vi "selectHotLotNewLinked.vi"() -> (0 "data":string, 3 "Array":string[][](array[string]))   [LabVIEW 2012]
uses:
  <vilib>/addons/database/Auxilliary.llb/DB Tools Cursor Type.ctl
  <vilib>/addons/database/Connection.llb/DB Tools Open Connec (Path).vi
  <vilib>/addons/database/Connection.llb/Conn Execute.vi
  <vilib>/addons/database/Recordset.llb/Rec Fetch Recordset Data (R).vi
  <vilib>/addons/database/Recordset.llb/Rec Destroy - Connection.vi
  <vilib>/addons/database/_DB Variant To Data/Database Variant To Data.xnode
  <vilib>/addons/database/NI_Database_API.lvlib
panel:
  in  "Cluster":T1
  out "data 2":string
  out "error out":errorcluster
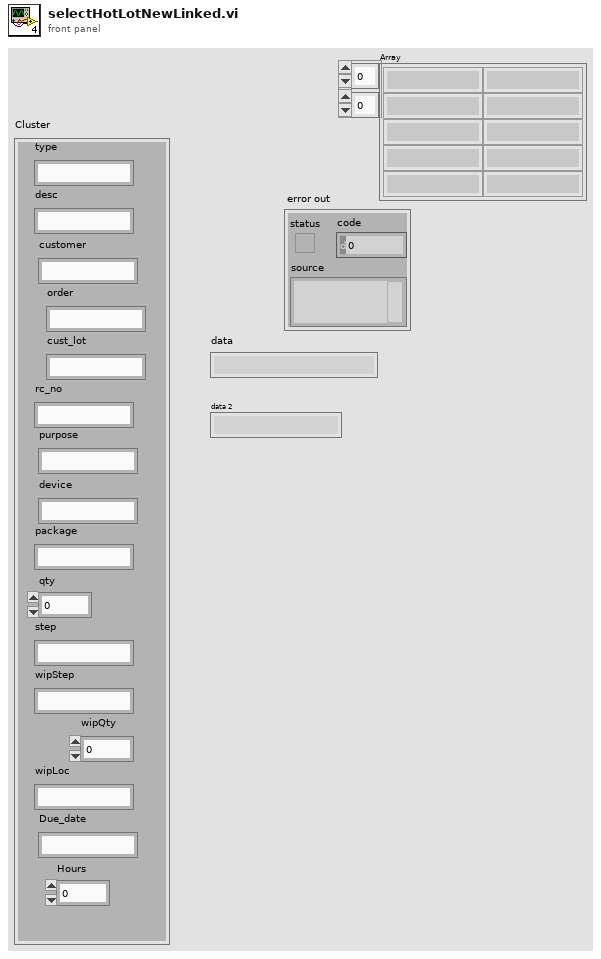
[diagram p1: front panel]
types:
  T1 = cluster{"type":string, "desc":string, "customer":string, "order":string, "cust_lot":string, "rc_no":string, "purpose":string, "device":string, "package":string, "qty":dbl, "step":string, "wipStep":string, "wipQty":dbl, "wipLoc":string, "Due_date":string, "Hours":dbl}
  T2 = typedef "NI_Database_API.lvlib/DB Tools Cursor Type.ctl" = enum16{"forward-only", "keyset", "dynamic", "static"}
  T3 = typedef "NI_Database_API.lvlib/Conn ObjectReference.ctl" = refnum<k1>
  T4 = typedef "NI_Database_API.lvlib/Rec ObjectReference.ctl" = refnum<k1>
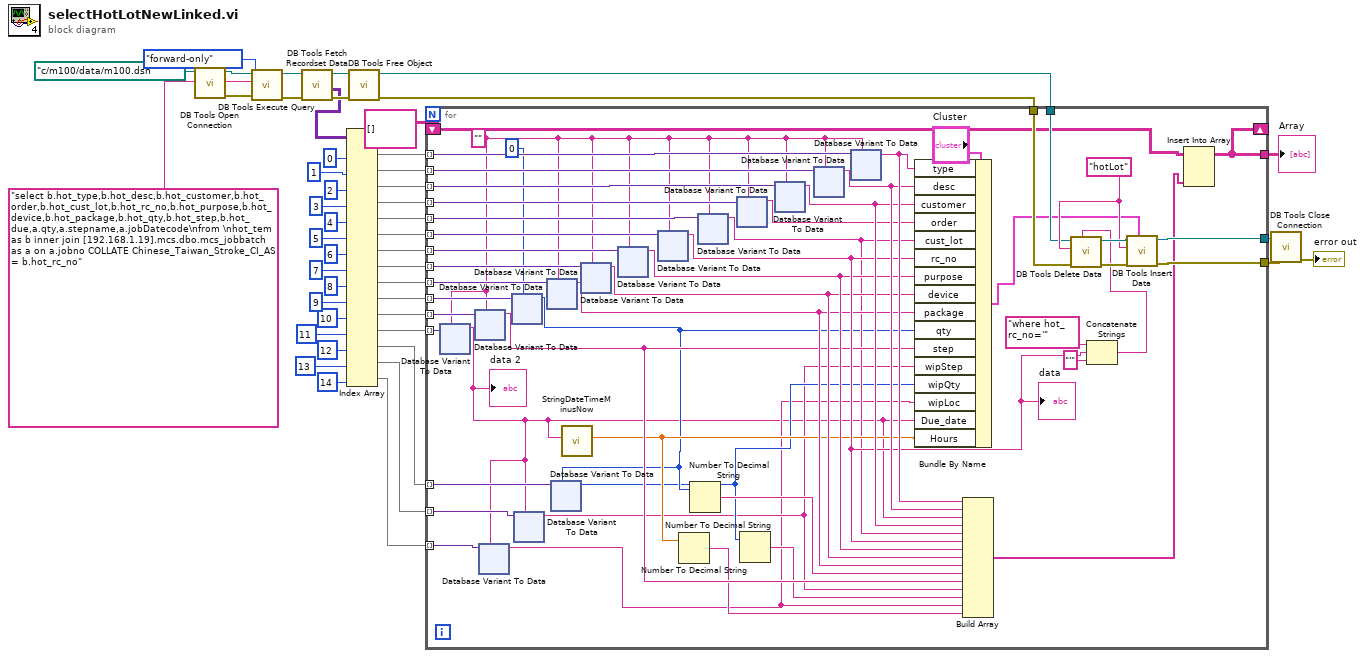
[diagram p0: block diagram]
diagram:
  n1 = call-poly <vilib>:"DB Tools Open Connection.vi"("connection information"=path "c:/m100/data/m100.dsn") -> ("error out"=w12:errorcluster, "connection reference"=w13:T3)  [unwired: 7 in]
  n2 = call-poly <vilib>:"DB Tools Execute Query.vi"("error in (no error)"=w12, "cursor type"=DB_Tools_Cursor_Type."forward-only", "SQL query"="select b.hot_type,b.hot_desc,b.hot_customer,b.hot_order,b.hot_cust_lot,b.hot_rc_no,b.hot_purpose,b.hot_device,b.hot_package,b.hot_qty,b.hot_step,b.hot_due,a.qty,a.stepname,a.jobDatecode\nfrom \nhot_tem as b inner join [192.168.1.19].mcs.dbo.mcs_jobbatch as a on a.jobno COLLATE Chinese_Taiwan_Stroke_CI_AS = b.hot_rc_no", "connection reference"=w13) -> ("error out"=w17:errorcluster, "recordset reference"=w16:T4)  [unwired: 4 in]
  n3 = call-poly <vilib>:"DB Tools Fetch Recordset Data.vi"("error in (no error)"=w17, "recordset reference"=w16) -> ("error out"=w15:errorcluster, "recordset data"=w9:variant[][], "recordset reference out"=w14:T4)  [unwired: 3 in]
  n4 = Index Array(array=w9, index (col) #1=0 ("disabled index (col)"), index (col) #2=1 ("index (col)"), index (col) #3=2 ("index (col)"), index (col) #4=3 ("index (col)"), index (col) #5=4 ("index (col)"), index (col) #6=5 ("index (col)"), index (col) #7=6 ("index (col)"), index (col) #8=7 ("index (col)"), index (col) #9=8 ("index (col)"), index (col) #10=9 ("index (col)"), index (col) #11=10 ("index (col)"), index (col) #12=11 ("index (col)"), index (col) #13=12 ("index (col)"), index (col) #14=13 ("index (col)"), index (col) #15=14 ("index (col)")) -> (element #1=w34:variant[], element #2=w33:variant[], element #3=w32:variant[], element #4=w31:variant[], element #5=w30:variant[], element #6=w29:variant[], element #7=w28:variant[], element #8=w27:variant[], element #9=w26:variant[], element #10=w25:variant[], element #11=w24:variant[], element #12=w20:variant[], element #13=w3:variant[], element #14=w2:variant[], element #15=w1:variant[])  [unwired: 15 in]
  n5 = call-poly <vilib>:"DB Tools Free Object.vi"("error in (no error)"=w15, "recordset reference"=w14) -> ("error out"=w10:errorcluster, "connection reference"=w11:T3)  [unwired: 8 in]
  n6 = for {
    tunnel: w34 -> [w98] mode=indexing
    tunnel: w33 -> [w97] mode=indexing
    tunnel: w32 -> [w96] mode=indexing
    tunnel: w31 -> [w95] mode=indexing
    tunnel: w30 -> [w94] mode=indexing
    tunnel: w29 -> [w93] mode=indexing
    tunnel: w28 -> [w92] mode=indexing
    tunnel: w27 -> [w91] mode=indexing
    tunnel: w26 -> [w90] mode=indexing
    tunnel: w25 -> [w88] mode=indexing
    tunnel: w24 -> [w89] mode=indexing
    tunnel: w11 -> [w79]
    tunnel: w10 -> [w80]
    tunnel: [w85] -> w23
    tunnel: [w84] -> w22
    tunnel: w20 -> [w75] mode=indexing
    shift-right: [w71] -> _
    shift-left: string[][] [] -> [w72]
    tunnel: [w71] -> w18
    tunnel: w3 -> [w55] mode=indexing
    tunnel: w2 -> [w54] mode=indexing
    tunnel: w1 -> [w53] mode=indexing
    w81 = "hotLot" ("table")
    w74 = ""
    n7 = xnode "Database Variant To Data"("database variant"=w75, "type"=w74) -> ("data"=w48:string)  [unwired: 1 in, 1 out]
    "data 2" <- w48
    n8 = xnode "Database Variant To Data"("database variant"=w89, "type"=w74) -> ("data"=w61:string)  [unwired: 1 in, 1 out]
    n9 = xnode "Database Variant To Data"("database variant"=w53, "type"=w48) -> ("data"=w49:string)  [unwired: 1 in, 1 out]
    n10 = xnode "Database Variant To Data"("database variant"=w88, "type"=0) -> ("data"=w52:i32)  [unwired: 1 in, 1 out]
    n11 = xnode "Database Variant To Data"("database variant"=w54, "type"=w48) -> ("data"=w50:string)  [unwired: 1 in, 1 out]
    n12 = xnode "Database Variant To Data"("database variant"=w90, "type"=w74) -> ("data"=w63:string)  [unwired: 1 in, 1 out]
    n13 = xnode "Database Variant To Data"("database variant"=w55, "type"=w52) -> ("data"=w51:i32)  [unwired: 1 in, 1 out]
    n14 = call "StringDateTimeMinusNow.vi"("String DateTime"=w48) -> ("DateTime - Now"=w59:dbl)  [unwired: 10 in]
    n15 = xnode "Database Variant To Data"("database variant"=w91, "type"=w74) -> ("data"=w64:string)  [unwired: 1 in, 1 out]
    n16 = xnode "Database Variant To Data"("database variant"=w92, "type"=w74) -> ("data"=w65:string)  [unwired: 1 in, 1 out]
    n17 = xnode "Database Variant To Data"("database variant"=w93, "type"=w74) -> ("data"=w66:string)  [unwired: 1 in, 1 out]
    "data" <- w66
    n18 = Number To Decimal String(number=w59) -> (decimal integer string=w58:string)  [unwired: 1 in]
    n19 = Number To Decimal String(number=w52) -> (decimal integer string=w62:string)  [unwired: 1 in]
    n20 = xnode "Database Variant To Data"("database variant"=w94, "type"=w74) -> ("data"=w56:string)  [unwired: 1 in, 1 out]
    n21 = xnode "Database Variant To Data"("database variant"=w95, "type"=w74) -> ("data"=w67:string)  [unwired: 1 in, 1 out]
    n22 = Number To Decimal String(number=w51) -> (decimal integer string=w60:string)  [unwired: 1 in]
    n23 = xnode "Database Variant To Data"("database variant"=w96, "type"=w74) -> ("data"=w68:string)  [unwired: 1 in, 1 out]
    n24 = xnode "Database Variant To Data"("database variant"=w97, "type"=w74) -> ("data"=w69:string)  [unwired: 1 in, 1 out]
    n25 = xnode "Database Variant To Data"("database variant"=w98, "type"=w74) -> ("data"=w70:string)  [unwired: 1 in, 1 out]
    n26 = Bundle By Name(cluster="Cluster", "type"=w70, "desc"=w69, "customer"=w68, "order"=w67, "cust_lot"=w56, "rc_no"=w66, "purpose"=w65, "device"=w64, "package"=w63, "qty"=w52, "step"=w61, "wipStep"=w50, "wipQty"=w51, "wipLoc"=w49, "Due_date"=w48, "Hours"=w59) -> (w73:T1)
    n27 = Build Array(w70, w69, w48, w68, w56, w66, w65, w64, w63, w62, w61, w50, w60, w49, w58) -> (w57:string[])
    n28 = Concatenate Strings("where hot_rc_no='" ("string"), w66, "'" ("string")) -> (w76:string)
    n29 = call <vilib>:"DB Tools Delete Data.vi"("condition"=w76, "error in (no error)"=w80, "table"=w81, "connection reference"=w79) -> ("error out"=w82:errorcluster, "connection reference out"=w83:T3)  [unwired: 6 in]
    n30 = call <vilib>:"DB Tools Insert Data.vi"("data"=w73, "error in (no error)"=w82, "table"=w81, "connection reference"=w83) -> ("error out"=w84:errorcluster, "connection reference out"=w85:T3)  [unwired: 6 in]
    n31 = Insert Into Array(array=w72, new element=w57) -> (w71:string[][])  [unwired: 2 in]
  }
  "Array" <- w18
  n32 = call <vilib>:"DB Tools Close Connection.vi"("error in (no error)"=w22, "connection reference"=w23) -> ("error out"=→"error out":errorcluster)  [unwired: 5 in]
